vi "SignalLeveling.vi"(1 "Noise Variability":dbl, 2 "Signal Level":dbl) -> (0 "Waveform Chart":dbl(graph))   [LabVIEW 2015]
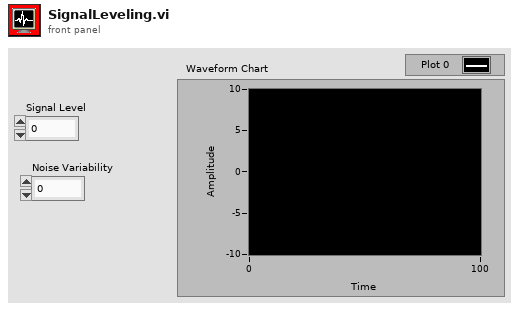
[diagram p1: front panel]
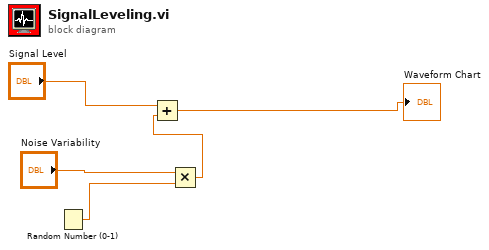
[diagram p0: block diagram]
diagram:
  n1 = Random Number (0-1)() -> (number: 0 to 1=w3:dbl)
  n2 = Multiply(x="Noise Variability", y=w3) -> (x*y=w2:dbl)
  n3 = Add(x="Signal Level", y=w2) -> (x+y=→"Waveform Chart":dbl)
